vi "Post Build.vi"(5 "Files Generated by Build":path[](array[path]), 6 "Top Level/Always Included VIs":path[](array[path]), 7 "Destination Path":path, 8 "error in (no error)":errorcluster, 9 "Target Name":string, 10 "Build Specification Name":string, 11 "Project Path":path) -> (0 "error out":errorcluster)   [LabVIEW 2015]
uses:
  <vilib>/AppBuilder/AB_API_Simple/Get Build Specification Version (path).vi
  <vilib>/AppBuilder/AB_API_Simple/NI_App_Builder_API.lvlib
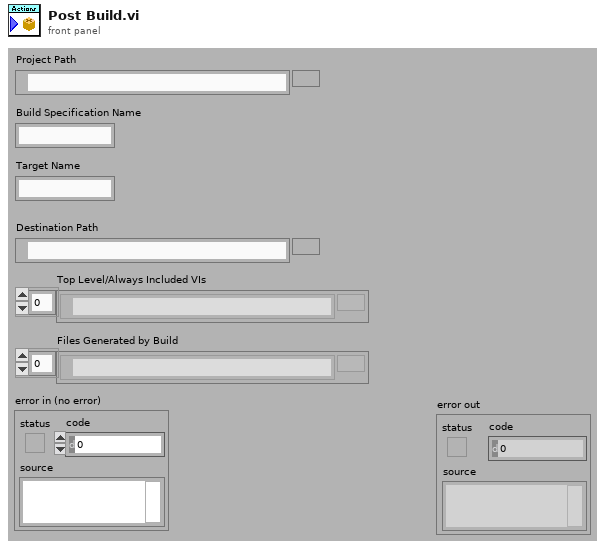
[diagram p1: front panel]
types:
  T1 = typedef "NI_App_Builder_API.lvlib/Build Specification Version.ctl" = cluster{"Major":u16, "Minor":u16, "Fix":u16, "Build":u16}
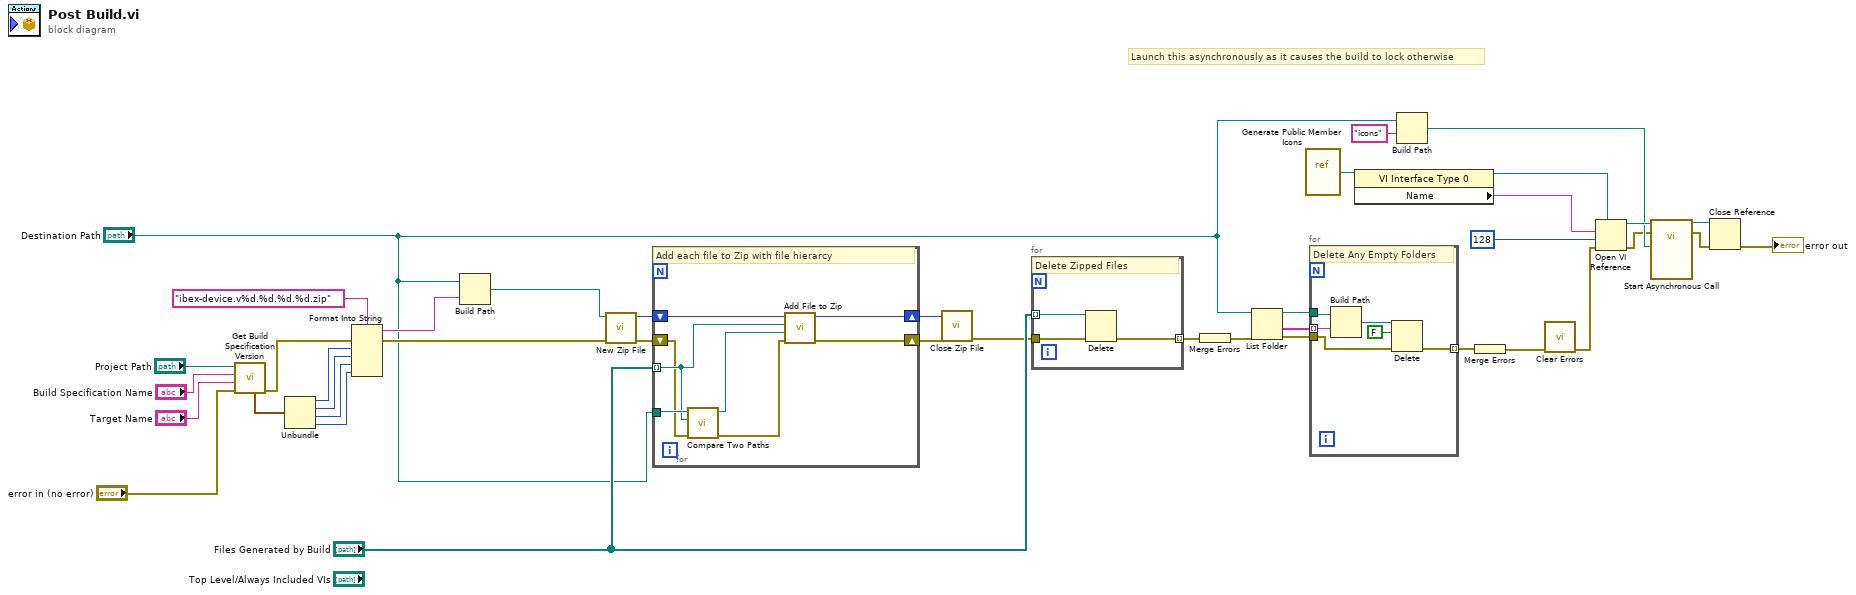
[diagram p0: block diagram]
diagram:
  # "Launch this asynchronously as it causes the build to lock otherwise"
  n1 = call-poly <vilib>:"Get Build Specification Version.vi"("error in (no error)"="error in (no error)", "Name of target (My Computer)"="Target Name", "Name of build specification"="Build Specification Name", "Path to project"="Project Path") -> ("error out"=w23:errorcluster, "Build Specification Version"=w37:T1)  [unwired: 6 in]
  n2 = Unbundle(w37) -> ("Major"=w36:u16, "Minor"=w35:u16, "Fix"=w34:u16, "Build"=w33:u16)
  n3 = Format Into String(format string="ibex-device.v%d.%d.%d.%d.zip", error in=w23, w36, w35, w34, w33) -> (resulting string=w30:string, error out=w31:errorcluster)  [unwired: 1 in]
  n4 = Build Path(base path="Destination Path", name or relative path=w30) -> (appended path=w29:path)
  n5 = call <vilib>:"New Zip File.vi"("error in (no error)"=w31, "target"=w29) -> ("error out"=w27:errorcluster, "zip file out"=w28:i64)  [unwired: 3 in, 1 out]
  n6 = for {
    tunnel: "Files Generated by Build" -> [w44] mode=indexing
    shift-right: [w46] -> w26
    shift-left: w27 -> [w43]
    shift-right: [w47] -> w25
    shift-left: w28 -> [w48]
    tunnel: "Destination Path" -> [w45]
    # "Add each file to Zip with file hierarcy"
    n7 = call <vilib>:"Compare Two Paths.vi"("error in (no error)"=w43, "Path 2"=w44, "Path 1"=w45) -> ("error out"=w41:errorcluster, "Relative Path from 1 to 2"=w42:path)  [unwired: 5 in, 2 out]
    n8 = call <vilib>:"Add File to Zip.vi"("error in (no error)"=w41, "destination path in zip"=w42, "source file path"=w44, "zip file in"=w48) -> ("error out"=w46:errorcluster, "zip file out"=w47:i64)  [unwired: 6 in]
  }
  n9 = call <vilib>:"Close Zip File.vi"("error in (no error)"=w26, "zip file in"=w25) -> ("error out"=w15:errorcluster)  [unwired: 5 in]
  n10 = for {
    tunnel: "Files Generated by Build" -> [w51] mode=indexing
    tunnel: [w50] -> w22 mode=indexing
    tunnel: w15 -> [w49]
    # "Delete Zipped Files"
    n11 = Delete(path (use dialog)=w51, error in=w49) -> (error out=w50:errorcluster)  [unwired: 3 in, 2 out]
  }
  n12 = Merge Errors(w22) -> (w21:errorcluster)
  n13 = List Folder(path="Destination Path", error in=w21) -> (path out=w18:path, folder names=w20:string[], error out=w19:errorcluster)  [unwired: 2 in, 1 out]
  n14 = vi-ref "Generate Public Member Icons.vi"() -> (w14:refnum<vi>)
  n15 = for {
    tunnel: w20 -> [w57] mode=indexing
    tunnel: w19 -> [w54]
    tunnel: w18 -> [w56]
    tunnel: [w52] -> w17 mode=indexing
    # "Delete Any Empty Folders"
    n16 = Build Path(base path=w56, name or relative path=w57) -> (appended path=w55:path)
    n17 = Delete(path (use dialog)=w55, entire hierarchy (F)=FALSE, error in=w54) -> (error out=w52:errorcluster)  [unwired: 2 in, 2 out]
  }
  n18 = property class="VI Interface Type 0"(reference=w14) -> (reference out=w12:refnum<vi>, "Name"=w13:string)  [unwired: 1 in, 1 out]
  n19 = Build Path(base path="Destination Path", name or relative path="icons") -> (appended path=w5:path)
  n20 = Merge Errors(w17) -> (w8:errorcluster)
  n21 = call <vilib>:"Clear Errors.vi"("error in (no error)"=w8) -> ("error out"=w1:errorcluster)  [unwired: 5 in, 1 out]
  n22 = Open VI Reference(type specifier VI Refnum (for type only)=w12, vi path=w13, options=128, error in (no error)=w1) -> (vi reference=w11:refnum<vi>, error out=w4:errorcluster)  [unwired: 2 in]
  n23 = call-by-ref "Start Asynchronous Call"(reference=w11, error in=w4, "Icon Destination Path"=w5) -> (reference out=w10:refnum<vi>, error out=w9:errorcluster)  [unwired: 10 in, 1 out]
  n24 = Close Reference(reference=w10, error in (no error)=w9) -> (error out=→"error out":errorcluster)
